vi "WindowsProcesses.vi"(8 "error in (no error)":errorcluster) -> (0 "error out":errorcluster, 2 "ProcessNames":string[](array[string]), 3 "WindowTitles":string[](array[string]))   [LabVIEW 2023]
doc: "Returns WindowTitles and lower case(!) ProcessNames of all running Processes\n\ninfo@becker-hickl.com"
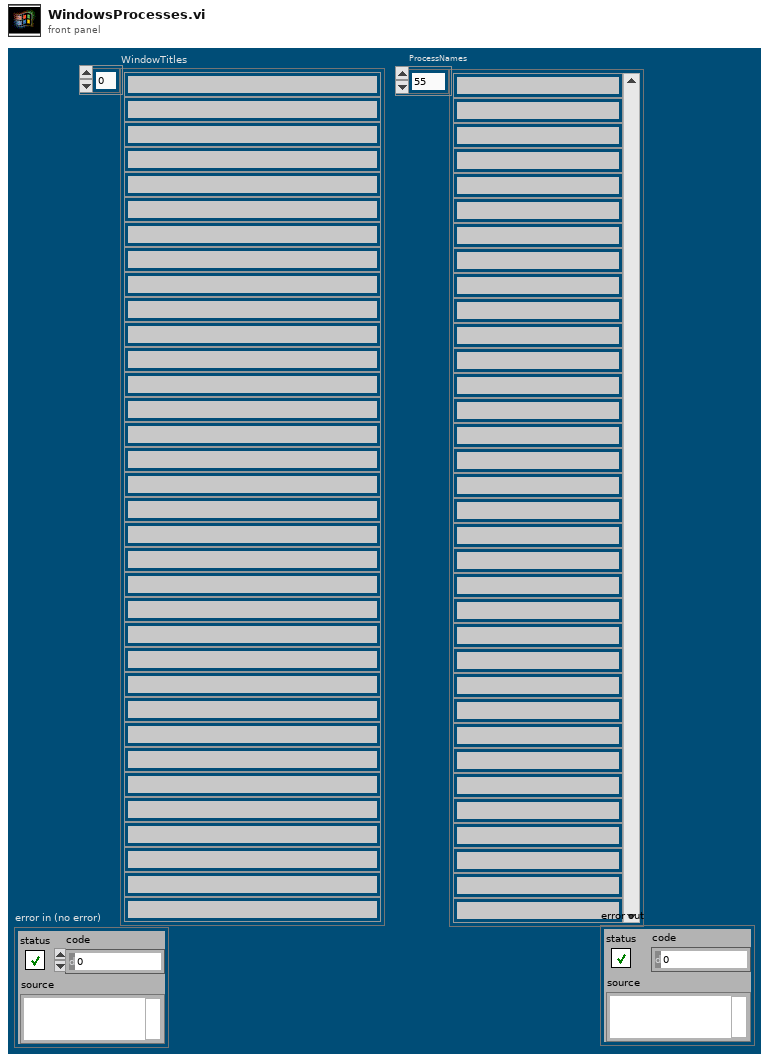
[diagram p1: front panel]
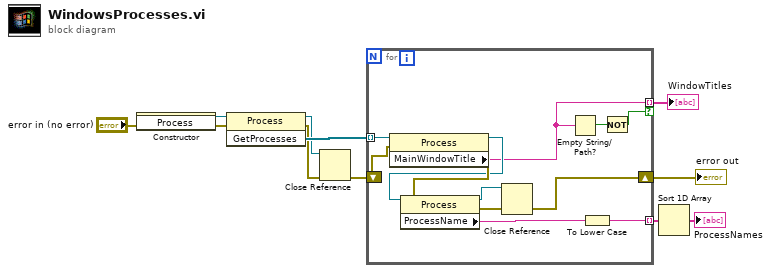
[diagram p0: block diagram]
diagram:
  n1 = constructor class="Process"(error in="error in (no error)") -> (reference out=w11:refnum<k24>, error out=w6:errorcluster)  [unwired: 2 in, 1 out]
  n2 = invoke class="Process" method="GetProcesses"(reference=w11, error in=w6) -> (reference out=w5:refnum<k24>, error out=w4:errorcluster, "GetProcesses"=w10:refnum<k24>[])  [unwired: 1 in]
  n3 = Close Reference(reference=w5, error in (no error)=w4) -> (error out=w3:errorcluster)
  n4 = for {
    tunnel: w10 -> [w18] mode=indexing
    tunnel: [w12] -> w8 mode=indexing
    shift-right: [w20] -> w2
    shift-left: w3 -> [w22]
    tunnel: [w16] -> w9 mode=indexing if=w14
    n5 = property class="Process"(reference=w18, error in=w22) -> (reference out=w17:refnum<k24>, error out=w21:errorcluster, "MainWindowTitle"=w16:string)
    n6 = property class="Process"(reference=w17, error in=w21) -> (reference out=w19:refnum<k24>, error out=w20:errorcluster, "ProcessName"=w13:string)
    n7 = Close Reference(reference=w19) -> ()  [unwired: 1 in, 1 out]
    n8 = Empty String/Path?(string/path=w16) -> (empty?=w15:bool)
    n9 = To Lower Case(string=w13) -> (all lower case string=w12:string)
    n10 = Not(x=w15) -> (.not. x?=w14:bool)
  }
  "WindowTitles" <- w9
  "error out" <- w2
  n11 = Sort 1D Array(array=w8) -> (sorted array=→"ProcessNames":string[])
